vi "索引脉冲(保持时间).vi"(8 "显示数据":i32[](array[numeric]), 10 "索引":i32, 11 "数据":T1[](array[typedef])) -> (0 "数组":T2[](array[typedef]), 3 "测试数据":T1)   [LabVIEW 2020]
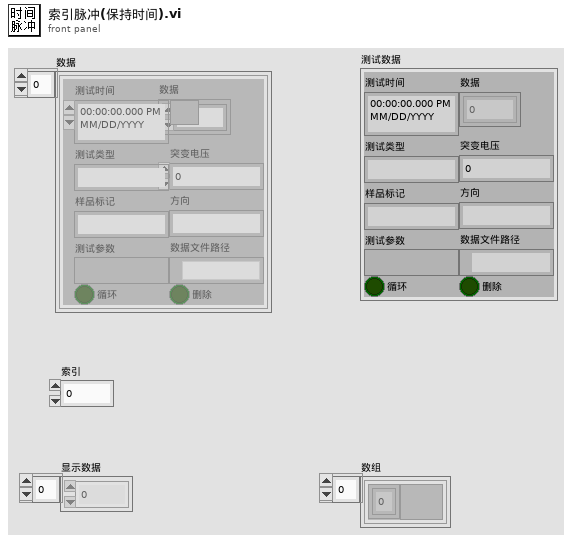
[diagram p1: front panel]
types:
  T1 = typedef "测试数据类型.ctl" = cluster{"测试时间":timestamp, "测试类型":string, "样品标记":string, "测试参数":variant, "循环":bool, "数据":dbl[][], "删除":bool, "突变电压":i32, "方向":string, "数据文件路径":path}
  T2 = typedef "数据显示.xctl/波形数据定义.ctl" = cluster{"波形":dbl[][], "属性":variant}
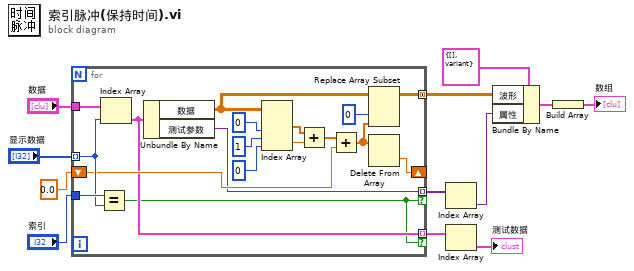
[diagram p0: block diagram]
diagram:
  n1 = for {
    tunnel: "显示数据" -> [w28] mode=indexing
    tunnel: "数据" -> [w30]
    tunnel: "索引" -> [w29]
    shift-right: [w25] -> _
    shift-left: 0.0 -> [w22]
    tunnel: [w13] -> w2 mode=indexing if=w15
    tunnel: [w16] -> w11 mode=indexing if=w15
    tunnel: [w14] -> w6 mode=concatenating
    n2 = Equal?(x=w29, y=w28) -> (x = y?=w15:bool)
    n3 = Index Array(array=w30, index=w28) -> (element=w16:T1)
    n4 = Unbundle By Name(w16) -> ("数据"=w27:dbl[][], "测试参数"=w13:variant)
    n5 = Index Array(array=w27, index (col) #1=0 ("索引 (行)"), index (row) #2=1 ("禁用的索引 (行)"), index (col) #2=0 ("索引 (列)")) -> (element #1=w23:dbl[], element #2=w17:dbl)  [unwired: 1 in]
    n6 = Add(x=w23, y=w17) -> (x+y=w18:dbl[])
    n7 = Add(x=w18, y=w22) -> (x+y=w21:dbl[])
    n8 = Replace Array Subset(array=w27, new element=w21, index (col)=0 ("禁用的索引 (列)")) -> (w14:dbl[][])  [unwired: 1 in]
    n9 = Delete From Array(array=w21) -> (deleted portion=w25:dbl)  [unwired: 2 in, 1 out]
  }
  n10 = Index Array(array=w2) -> (element=w1:variant)  [unwired: 1 in]
  n11 = Index Array(array=w11) -> (element=→"测试数据":T1)  [unwired: 1 in]
  n12 = Bundle By Name(cluster=T2 {"波形"=[], "属性"=variant} ("波形数据"), "波形"=w6, "属性"=w1) -> (w5:T2)
  n13 = Build Array(w5) -> (→"数组":T2[])
